vi "[Global]iVision_Version.vi"() -> ()   [LabVIEW 2019]
panel:
  in  "iVision_Version":string
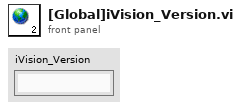
[diagram p1: front panel]
diagram:
